vi "Determine Warning - Temperature and Wind subVIs.vi"(6 "강풍":dbl, 7 "현재 풍속":dbl, 8 "에러 입력 (에러 없음)":errorcluster caption="에러 입력(에러 없음)", 9 "최저 온도":dbl, 10 "최고 온도":dbl, 11 "현재 온도":dbl) -> (0 "에러 출력":errorcluster, 1 "경고?":bool, 2 "경고 텍스트":string)   [LabVIEW 2010]
doc: "이 VI는 LabVIEW Core II 교육 과정의 연습문제에 대한 해답입니다. 이 연습문제에서는 상속받은 코드를 가지고 읽기 쉽고 관리하기 쉽게 만듭니다."
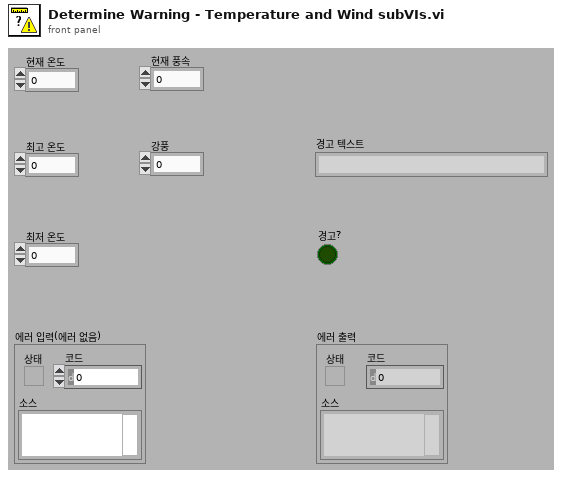
[diagram p1: front panel]
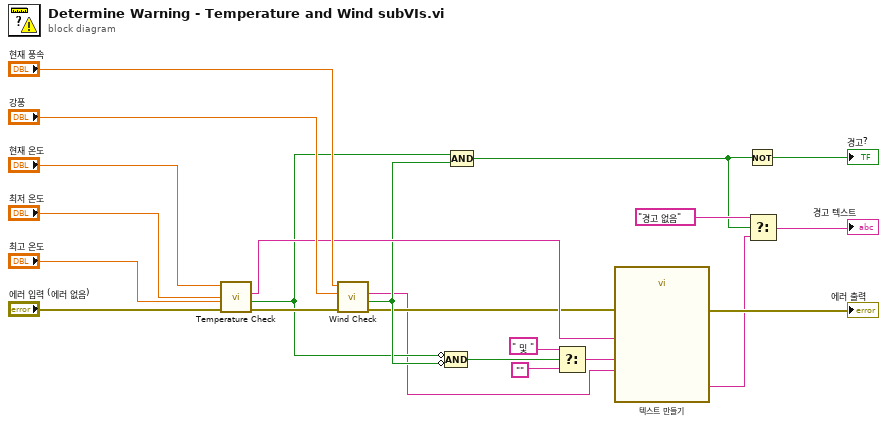
[diagram p0: block diagram]
diagram:
  n1 = call "Temperature Check.vi"("에러 입력 (에러 없음)"="에러 입력 (에러 없음)", "고온"="최고 온도", "저온"="최저 온도", "현재 온도"="현재 온도") -> ("에러 출력"=w5:errorcluster, "온도 경고?"=w3:bool, "온도 경고"=w13:string)  [unwired: 5 out]
  n2 = call "Wind Check.vi"("에러 입력(에러 없음)"=w5, "강풍"="강풍", "현재 풍속"="현재 풍속") -> ("에러 출력"=w2:errorcluster, "풍속 경고?"=w4:bool, "풍속 경소 메시지"=w1:string)  [unwired: 6 out]
  n3 = Compound Arithmetic op=AND(invert w3, invert w4) -> (w7:bool)
  n4 = Compound Arithmetic op=AND(w3, w4) -> (w6:bool)
  n5 = Select(t=" 및 ", s=w7, f="") -> (s? t:f=w11:string)
  n6 = call "텍스트 만들기"("온도 경고"=w13, "및"=w11, "동상 경고"=w1, "error in (no error)"=w2) -> ("Result"=w8:string, "error out"=→"에러 출력":errorcluster)  [unwired: 1 in, 9 out]
  n7 = Not(x=w6) -> (.not. x?=→"경고?":bool)
  n8 = Select(t="경고 없음", s=w6, f=w8) -> (s? t:f=→"경고 텍스트":string)
